vi "Remove Module.vi"(0 "BroadcastRegistry In":T1, 7 "Source":string) -> (4 "BroadcastRegistry Out":T1)   [LabVIEW 2017, in "Communicable State Machine.lvlib"]
doc: "### Remove Module.vi\n\n-- <b>Controls</b> --\n- <b>BroadcastRegistry in</b>:\n- <b>Source</b>:\n\n-- <b>Indicators</b> --\n- <b>BroadcastRegistry out</b>:"
uses:
  Communicable State Machine.lvlib
  BroadcastRegistry.ctl
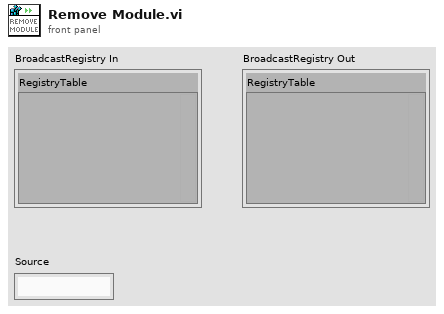
[diagram p1: front panel]
types:
  T1 = typedef "Communicable State Machine.lvlib/BroadcastRegistry.ctl" = cluster{"RegistryTable":variant}
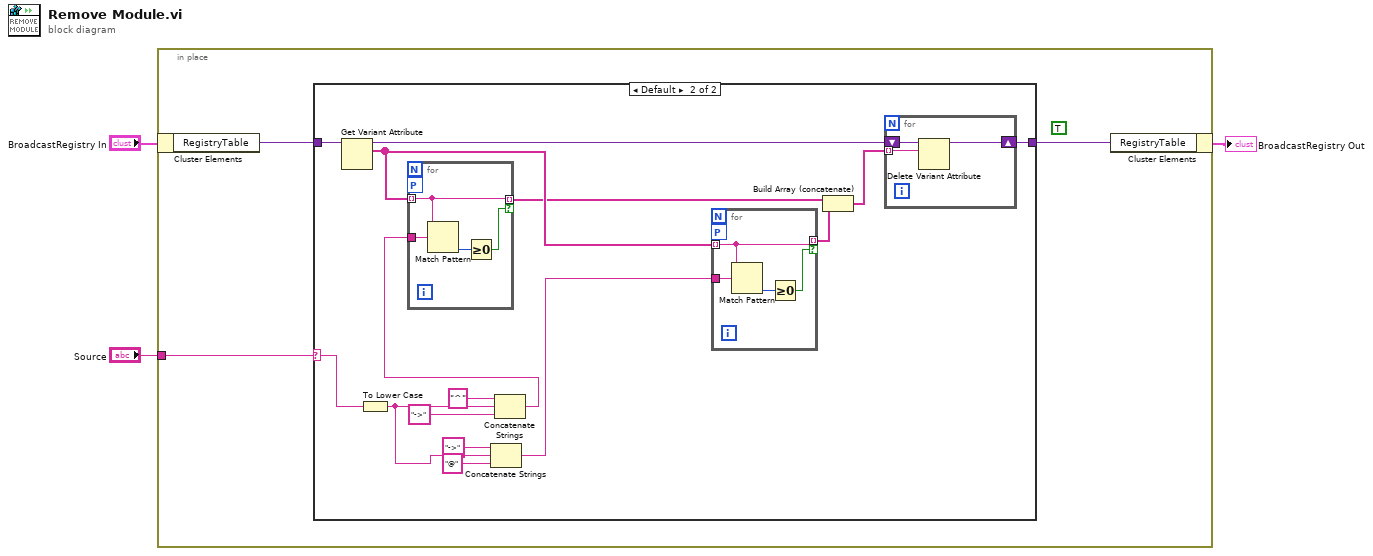
[diagram p0: block diagram]
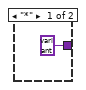
[diagram p2: hidden frame]
diagram:
  n1 = in-place {
    in-place-border: "Source" -> [w4]
    (unwired) TRUE ("Cache changed?")
    n2 = in-place-cluster #1("BroadcastRegistry In") -> ("RegistryTable"=w6:variant)
    n3 = case shown="Default" w4 {
      selector: w4 -> [_ w8]
      tunnel: [variant w21] -> w5
      tunnel: w6 -> [_ w20]
      frame "*" {
      }
      frame Default {
        n4 = Get Variant Attribute(Variant=w20) -> (duplicate Variant=w19:variant, names=w16:string[])  [unwired: 3 in, 2 out]
        n5 = To Lower Case(string=w8) -> (all lower case string=w13:string)
        n6 = Concatenate Strings("->" ("string"), w13, "@" ("string")) -> (w11:string)
        n7 = Concatenate Strings("^" ("string"), w13, "->" ("string")) -> (w12:string)
        n8 = for {
          tunnel: w16 -> [w26] mode=indexing
          tunnel: [w26] -> w9 mode=indexing if=w24
          tunnel: w12 -> [w23]
          workers-P: _ -> [_]
          n9 = Match Pattern(string=w26, regular expression=w23) -> (offset past match=w25:i32)  [unwired: 1 in, 3 out]
          n10 = Greater Or Equal To 0?(x=w25) -> (x >= 0?=w24:bool)
        }
        n11 = for {
          tunnel: w16 -> [w33] mode=indexing
          tunnel: [w33] -> w18 mode=indexing if=w30
          tunnel: w11 -> [w32]
          workers-P: _ -> [_]
          n12 = Match Pattern(string=w33, regular expression=w32) -> (offset past match=w31:i32)  [unwired: 1 in, 3 out]
          n13 = Greater Or Equal To 0?(x=w31) -> (x >= 0?=w30:bool)
        }
        n14 = Build Array (concatenate)(w9, w18) -> (w10:string[])
        n15 = for {
          tunnel: w10 -> [w27] mode=indexing
          shift-right: [w29] -> w21
          shift-left: w19 -> [w28]
          n16 = Delete Variant Attribute(6:w27, 7:w28) -> (3:w29:variant)  [unwired: 1 in, 2 out]
        }
      }
    }
    n17 = in-place-cluster #1("RegistryTable"=w5) -> (→"BroadcastRegistry Out":T1)
  }
